vi "Create AnalogInput DAQmx(PhysChannel).vi"(5 "Subsystem in":refnum<class "DAQmx(AI).lvclass">, 6 "Input Configuration":T1={"input terminal"=10083, "minimum value"=-5.0, "maximum value"=5.0, "units"=enum."Volts"} {"maximum value" format="%#_13g"; "minimum value" format="%#_13g"; "input terminal" items=["Default"=-1, "RSE"=10083, "NRSE"=10078, "Differential"=10106, "Pseudodifferential"=12529]}, 7 "task name":string, 8 "error in (no error)":errorcluster, 9 "Period (ms)":i64=50, 10 "Subsystem Name (optional)":string, 11 "DAQmx Physical Channel":tag) -> (0 "error out":errorcluster, 2 "SMO name":string, 3 "Subsystem out":refnum<class "DAQmx(AI).lvclass">)   [LabVIEW 2013, in "DAQmx(AI).lvclass"]
uses:
  DAQmx(AI).lvclass
  Typedefs/InputConfiguration--Cluster.ctl
  Typedefs/Units -- Enum.ctl
  Typedefs/Configuration--Cluster.ctl
  <vilib>/JKI/JKI SMO/SMO/SMO.lvclass
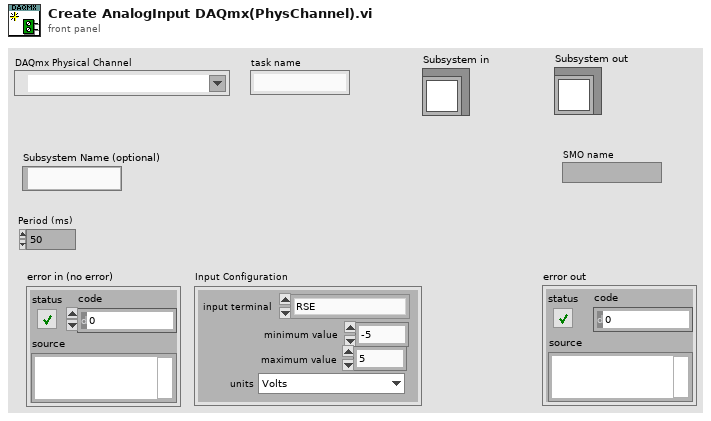
[diagram p1: front panel]
types:
  T1 = typedef "DAQmx(AI).lvclass/InputConfiguration--Cluster.ctl" = cluster{"input terminal":i32, "minimum value":dbl, "maximum value":dbl, "units":T2}
  T2 = typedef "DAQmx(AI).lvclass/Units -- Enum.ctl" = enum16{"Volts", "Amps", "Deg F", "Deg C", "Deg R", "Kelvins", "Strain", "Ohms", "Hz", "Seconds", "Meters", "Inches", "Degrees", "Radians", "Ticks", "g", "m/s^2", "m/s", "in/s", "Pascals", "Newtons", "Pounds", "kgf", "psi", "bar", "Nm", "oz-in", "lb-in", "lb-ft", "Volts/Volt", "mVolts/Volt", "From TEDS"}
  T3 = typedef "DAQmx(AI).lvclass/Configuration--Cluster.ctl" = cluster{"PhysChan":tag, "Period (ms)":i64, "input terminal cfg":i32, "minimum value":dbl, "maximum value":dbl, "units":T2, "task name":string}
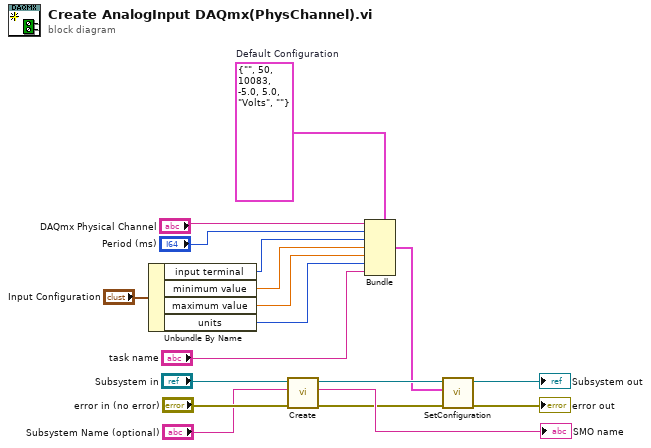
[diagram p0: block diagram]
diagram:
  w7 = T3 {"PhysChan"="", "Period (ms)"=50, "input terminal cfg"=10083, "minimum value"=-5.0, "maximum value"=5.0, "units"=enum."Volts", "task name"=""}  # Default Configuration
  n1 = Unbundle By Name("Input Configuration") -> ("input terminal"=w5:i32, "minimum value"=w4:dbl, "maximum value"=w3:dbl, "units"=w2:T2)
  n2 = call <vilib>:"Create.vi"("error in (no error)"="error in (no error)", "Subsystem Name (optional)"="Subsystem Name (optional)", "SMO"="Subsystem in") -> ("error out"=w14:errorcluster, "SMO name"=→"SMO name":string, "SMO out"=w12:refnum<class "DAQmx(AI).lvclass">)  [unwired: 6 in]
  n3 = Bundle(cluster=w7, "PhysChan"="DAQmx Physical Channel", "Period (ms)"="Period (ms)", "input terminal cfg"=w5, "minimum value"=w4, "maximum value"=w3, "units"=w2, "task name"="task name") -> (w9:T3)
  n4 = call "SetConfiguration.vi"("error in (no error)"=w14, "Configuration"=w9, "Subsystem"=w12) -> ("error out"=→"error out":errorcluster, "Subsystem out"=→"Subsystem out":refnum<class "DAQmx(AI).lvclass">)  [unwired: 7 in]
